vi "mainStationMeteo.vi"() -> ()   [LabVIEW 2017]
panel:
  out "sortie d'erreur":errorcluster caption="CLUSTER d'erreur"
  in  "Set Start Time (s)":dbl caption="Définir l'intervale d'acquisition (s)"
  out "Valeurs en temps réel":string
  in  "Bouton OK":bool
  out "Alarme":bool
  out "Etat":T1(ring)
  in  "?":bool
  # "Station Météo"
  # "BENOIT MANGEARD | JIXIONG LIU - 2018"
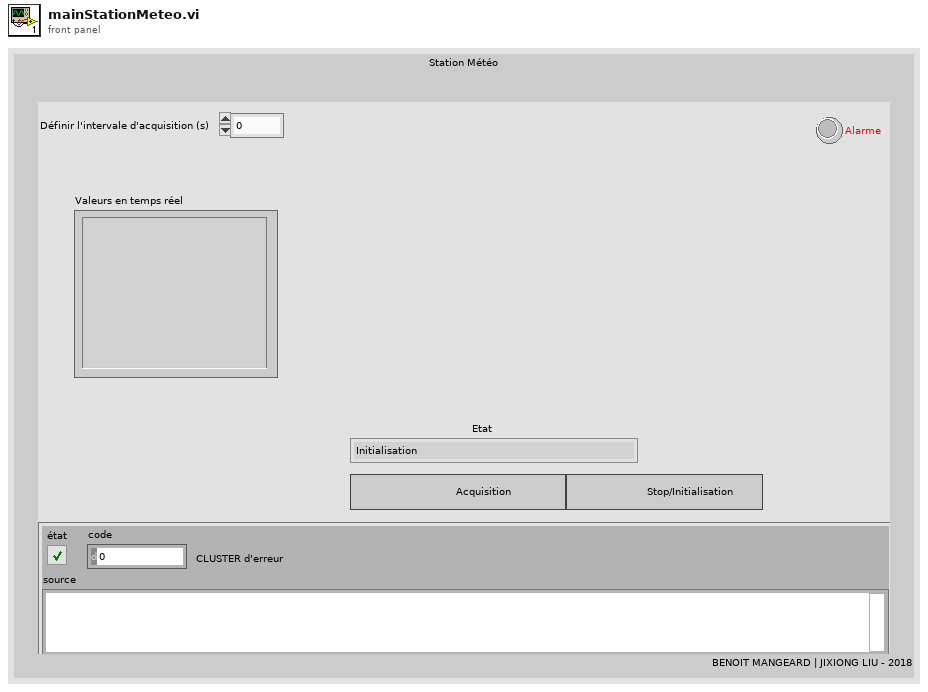
[diagram p1: front panel]
types:
  T1 = enum16{"Initialisation", "Acquisition", "Analyse", "Enregistrer", "Vérification du temps et Stop", "Fin"}
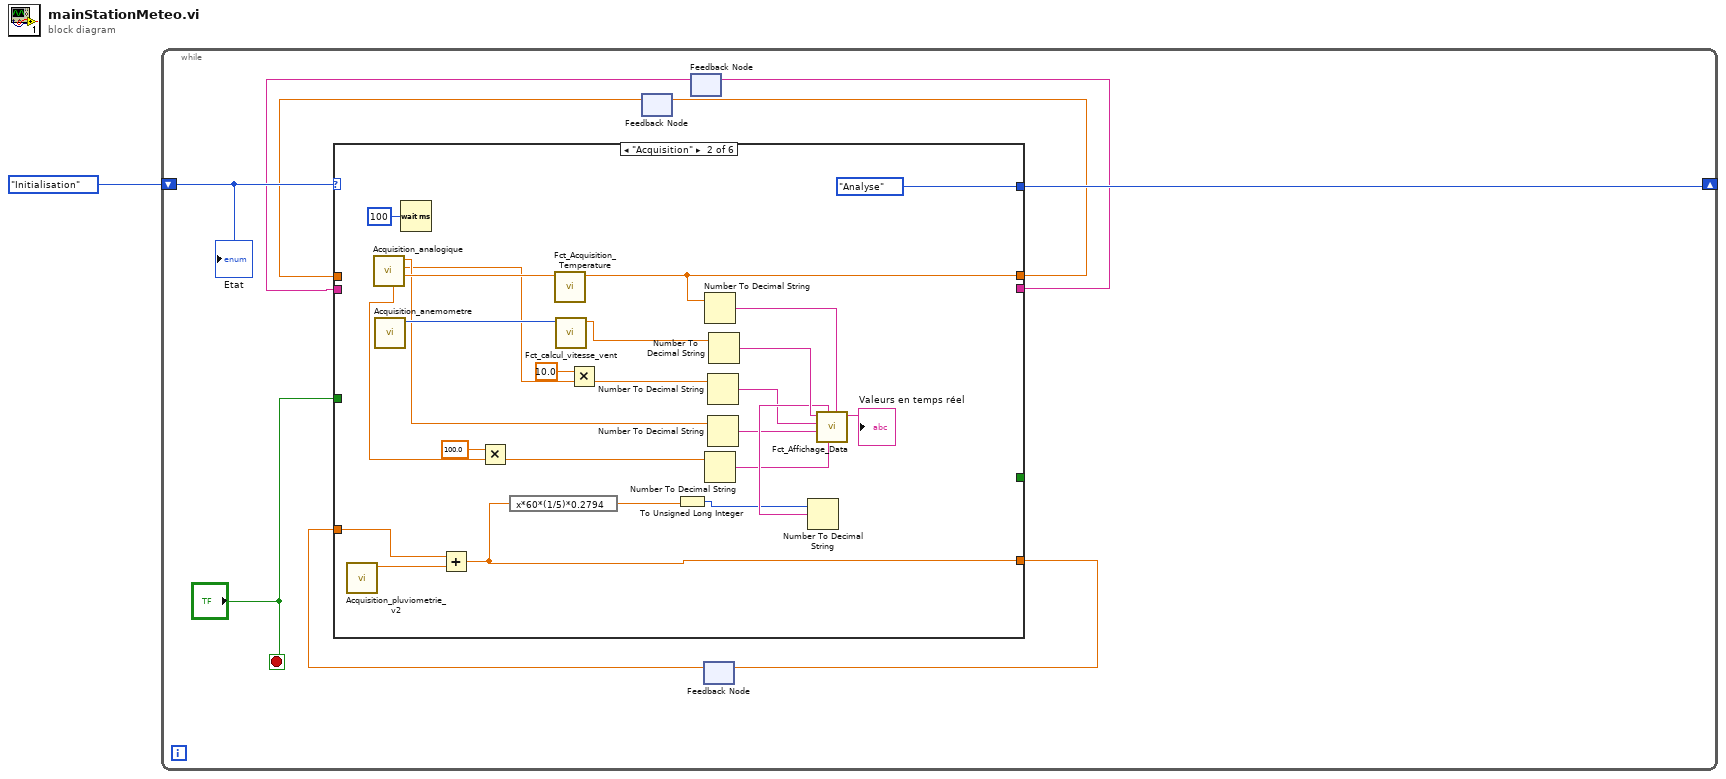
[diagram p0: block diagram]
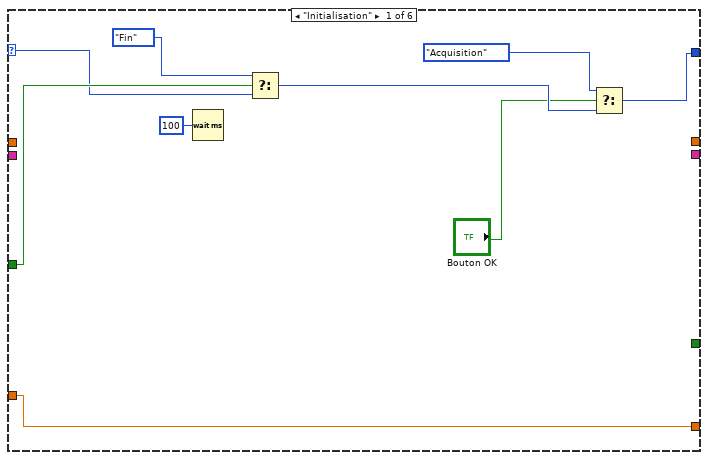
[diagram p2: hidden frame]
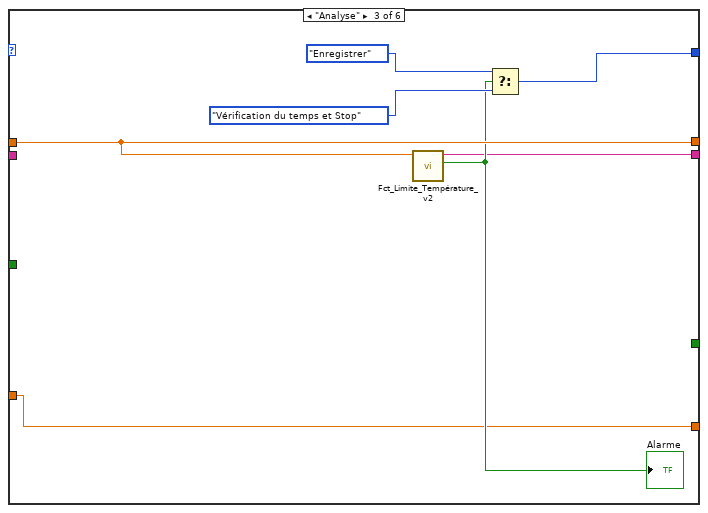
[diagram p3: hidden frame]
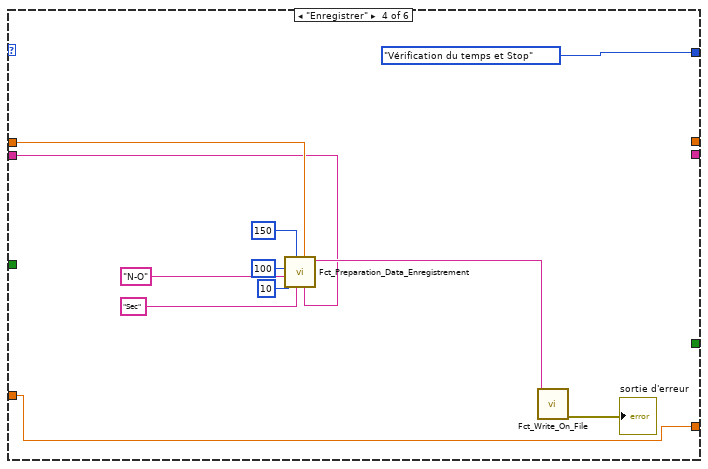
[diagram p4: hidden frame]
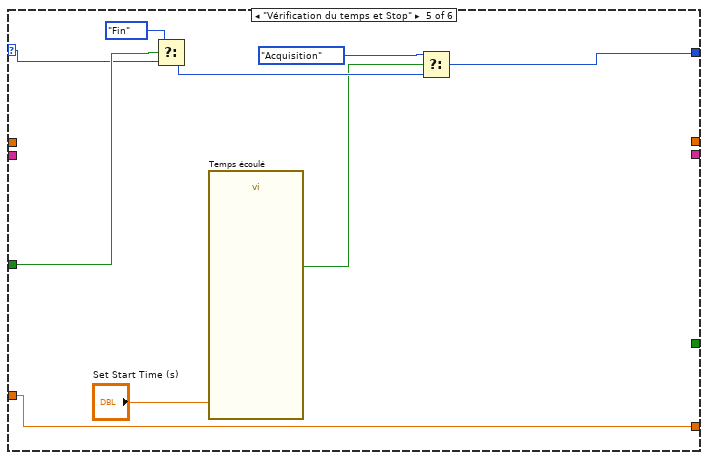
[diagram p5: hidden frame]
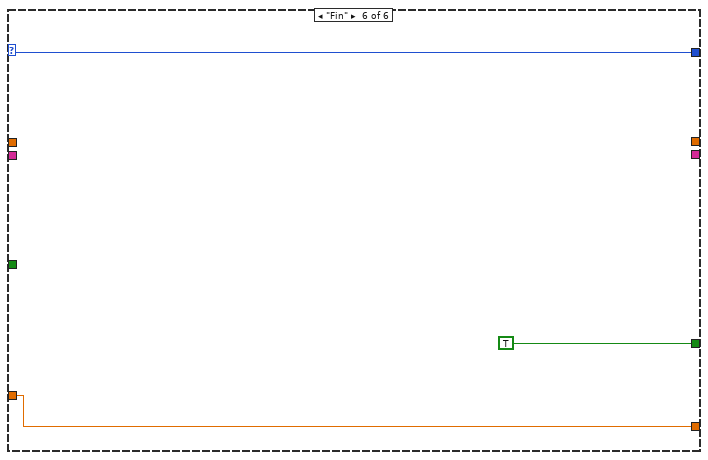
[diagram p6: hidden frame]
diagram:
  n1 = while {
    shift-right: [w10] -> _
    shift-left: T1."Initialisation" -> [w8]
    stop <- "?" stop-if-true
    n2 = feedback #1() -> (w6:dbl)  [unwired: 1 in]
    n3 = feedback #2() -> (w4:string)  [unwired: 1 in]
    n4 = feedback #3() -> (w2:dbl)  [unwired: 1 in]
    n5 = case "Structure Condition" shown="\"Acquisition\"" w8 {
      selector: w8 -> [w17 _ _ _ w65 w74]
      tunnel: [w13 T1."Analyse" w49 T1."Vérification du temps et Stop" w71 w74] -> w10
      tunnel: "?" -> [w18 _ _ _ w68 _]
      tunnel: [_ _ _ _ _ TRUE] -> _
      tunnel: [_ w40 w48 _ _ _] -> w7
      tunnel: w6 -> [_ _ w48 w59 _ _]
      tunnel: [_ _ w46 _ _ _] -> w5
      tunnel: w4 -> [_ _ _ w57 _ _]
      tunnel: [w11 w32 w45 w52 w63 w72] -> w3
      tunnel: w2 -> [w11 w33 w45 w52 w63 w72]
      frame "Initialisation" {
        n6 = Wait (ms)(milliseconds to wait=u32 100 ("attente (ms)")) -> ()  [unwired: 1 out]
        n7 = Select(t=T1."Fin", s=w18, f=w17) -> (s? t:f=w15:T1)
        n8 = Select(t=T1."Acquisition", s="Bouton OK", f=w15) -> (s? t:f=w13:T1)
      }
      frame "Acquisition" {
        n9 = call "Acquisition_pluviometrie_v2.vi"() -> ("Numérique"=w34:dbl)  [unwired: 11 in]
        n10 = call "Acquisition_analogique.vi"() -> ("Température"=w39:dbl, "Girouette"=w20:dbl, "Humidité"=w21:dbl, "Lumière"=w29:dbl)  [unwired: 8 in]
        n11 = call "Acquisition_anemometre.vi"() -> ("data"=w37:u32)  [unwired: 11 in]
        n12 = Wait (ms)(milliseconds to wait=u32 100 ("attente (ms)")) -> ()  [unwired: 1 out]
        n13 = Add(x=w33, y=w34) -> (x+y=w32:dbl)
        n14 = Multiply(x=100.0, y=w29) -> (x*y=w25:dbl)
        n15 = expression code="x*60*(1/5)*0.2794"(w32) -> (w31:dbl)
        n16 = call "Fct_Acquisition_Temperature.vi"("Tension"=w39) -> ("Température"=w40:dbl)  [unwired: 7 in, 3 out]
        n17 = call "Fct_calcul_vitesse_vent.vi"("data"=w37) -> ("Vent"=w36:dbl)  [unwired: 10 in]
        n18 = Multiply(x=10.0, y=w20) -> (x*y=w23:dbl)
        n19 = To Unsigned Long Integer(number=w31) -> (unsigned 32bit integer=w30:u32)
        n20 = Number To Decimal String(number=w40) -> (decimal integer string=w41:string)  [unwired: 1 in]
        n21 = Number To Decimal String(number=w25) -> (decimal integer string=w28:string)  [unwired: 1 in]
        n22 = Number To Decimal String(number=w23) -> (decimal integer string=w26:string)  [unwired: 1 in]
        n23 = Number To Decimal String(number=w21) -> (decimal integer string=w27:string)  [unwired: 1 in]
        n24 = Number To Decimal String(number=w36) -> (decimal integer string=w38:string)  [unwired: 1 in]
        n25 = Number To Decimal String(number=w30) -> (decimal integer string=w35:string)  [unwired: 1 in]
        n26 = call "Fct_Affichage_Data.vi"("Température"=w41, "Luminosité"=w28, "Pluiviométrie"=w35, "Humidité"=w27, "Direction du vent"=w26, "Vitesse vent"=w38) -> ("Sortie"=→"Valeurs en temps réel":string)  [unwired: 5 in]
      }
      frame "Analyse" {
        n27 = call "Fct_Limite_Température_v2.vi"("Température"=w48) -> ("Booléen"=w47:bool, "Chaîne"=w46:string)  [unwired: 9 in]
        "Alarme" <- w47
        n28 = Select(t=T1."Enregistrer", s=w47, f=T1."Vérification du temps et Stop") -> (s? t:f=w49:T1)
      }
      frame "Enregistrer" {
        n29 = call "Fct_Preparation_Data_Enregistrement.vi"("Motif"=w57, "Temperature"=w59, "Humidité"="Sec", "Vitesse vent"=150, "Direction Vent"="N-O", "Luminosité"=100, "Précipitation"=10) -> ("Chaîne"=w60:string)  [unwired: 4 in]
        n30 = call "Fct_Write_On_File.vi"("Chaîne"=w60) -> ("sortie d'erreur"=→"sortie d'erreur":errorcluster)  [unwired: 10 in]
      }
      frame "Vérification du temps et Stop" {
        n31 = Select(t=T1."Fin", s=w68, f=w65) -> (s? t:f=w66:T1)
        n32 = call "Temps écoulé"("Time Target (s)"="Set Start Time (s)") -> ("Time has Elapsed"=w64:bool)  [unwired: 11 in, 7 out]
        n33 = Select(t=T1."Acquisition", s=w64, f=w66) -> (s? t:f=w71:T1)
      }
      frame "Fin" {
      }
    }
    n34 = feedback-in #1(w7) -> ()
    n35 = feedback-in #2(w5) -> ()
    n36 = feedback-in #3(w3) -> ()
    "Etat" <- w8
  }
